vi "SYST_PRES.vi"(0 "VISA IN":refnum<visa-resource-name>, 5 "error in":errorcluster) -> (14 "VISA Out":refnum<visa-resource-name>, 19 "error out":errorcluster)   [LabVIEW 2018, in "PNA-X.lvlib"] (continued)
D6C-00108334AE96}\" \nQuery Syntax Not Applicable \nDefault Not Applicable \nSENSe:CORRection:COLLect:GUIDed:DMATch:APPLy:PORTs? \n1649\n\n(Read-only) Returns the port numbers for which delta match correction is required. 0 (zero) is \nreturned if the Cal does NOT require Delta Match correction for one of the following reasons: \nThe Cal does NOT involve Unknown THRU or TRL. You specify this using \nSENS:CORR:COLL:GUID:METH <UNKN | TRL>. \nThe Cal DOES involve Unknown THRU or TRL, but the delta match data can be calculated by the Unknown \nThru or TRL Cal. Learn how this is possible. However, you can force the Cal to use the Delta Match data \nfrom a Cal Set. \nLearn more about Delta match calibration. \nSee example of a complete Delta Match calibration. \nParameters \nExamples SENS:CORR:COLL:GUID:APPL:PORT? \n'Returns: \n1,2,3 \nReturn Type Numeric \nDefault Not Applicable \nSENSe:CORRection:COLLect:GUIDed:DMATch[:INITiate] <conn>,<cKit> \n(Write-only) Initiates a global delta match calibration. \nLearn more about Global Delta Match calibration. \nSee example of a complete Delta Match calibration. \nParameters \n<conn> String. Connector type for port 1. All other ports are set automatically. \n<cKit> String Cal Kit for all ports. If incorrectly entered while writing, an error is \nreturned. \nExamples SENS:CORR:COLL:GUID:DMAT APC 3.5 female,\"85052B\" \nQuery Syntax Not Applicable \nDefault Not Applicable \nSENSe:CORRection:COLLect:GUIDed:ETERms:LOAD[:CSET] <cset>,<calPort> [,csPort] \n1650\n\n(Write-only) Loads 1-port error terms from a Cal Set into the current Guided Cal sequence. When the \nCal steps are recomputed, connection steps are removed due to the loading of the error terms. \nSee example of how to use this command. \nParameters \n<cset> String Name of User Cal Set in which the error terms reside. \n<pnum> Integer Port number of the current cal to receive error terms. \n[csPort] Integer Optional argument. Port number associated with the error terms in the \nCal Set. If unspecified, the same port number as <calPort> is used. \nExamples See example \nQuery Syntax Not Applicable \nDefault Not Applicable \nSENSe<cnum>:CORRection:COLLect:GUIDed:INITiate [cal set name or GUID [,bool]] \n(Write-only) Initiates a guided calibration. \nThe PNA determines the measurements needed to perform the calibration using the settings specified from \nthe SENS:CORR:COLL:GUID:CONN:PORT and SENS:CORR:COLL:GUID:CKIT:PORT commands. \nAfter this command is executed, subsequent commands can be used to query the number of measurement \nsteps, issue the acquisition commands, query the connection description strings, and subsequently \ncomplete a guided calibration. \nParameters \n<cnum> Any existing channel number. If unspecified, value is set to 1 \n<cal set name or \nGUID> \n(String) Optional argument. If NOT specified, behavior depends on the \nSENS:CORR:PREFerence:CSET:SAVE setting. \nIf specified, choose an existing Cal Set, either by name or by GUID. \nCal Set name including quotes \nCalset GUID in the form: \"{GUID}\"; including quotes and curly brackets. \nQuery all Cal Set GUIDs with SENS:CORR:CSET:CAT? \nSENS:CORR:COLL:GUID:SAVE:CSET can be used instead of this optional \nargument to specify the GUID for a Cal Set. \nAn error is reported if the Cal Set is not found. \n1651\n\nThe Cal Set is either supplemented or overwritten depending on the method, \nconnectors, and ports selected. Learn more about Cal Sets. \n<bool> Optional argument. \nFalse (0) If Cal Set stimulus settings differ from the existing channel, do not \nchange channel stimulus settings. The Cal Set is save to the current setting of \nthe SENS:CORR:PREF:CSET:SAVE command. This is the default setting if \nnot specified. \nTrue (1) If cal set stimulus settings differ from the existing channel, change \nthe channel stimulus settings to match the Cal Set settings. \nExamples SENS:CORR:COLL:GUID:INIT \"{2B893E7A-971A-11d5-8D6C- \n00108334AE96}\",1 \nsense2:correction:collect:guided:initiate 'myCalSet' \nQuery Syntax Not Applicable \nDefault Not Applicable \nSENSe:CORRection:COLLect:GUIDed:ISOLation:AVERage:INCRement <num> \n(Read-Write) Specifies amount to increment (increase) the channel�s averaging factor during \nmeasurement of isolation standards in a guided calibration. \nNote: If the channel has averaging turned OFF and the value of <num> is greater than 1, averaging \nwill be turned ON only during the isolation measurements and with the averaging factor equal to \n<num>.\nParameters \n<num> Amount to increment the averaging factor for the isolation measurement. The \nmaximum averaging factor for the channel is 65536 (2^16). \nExamples 'Measure isolation on all paths for the cal \nSENS:CORR:COLL:GUID:ISOL ALL \n'Remove the port pairs 1-to-2 and 1-to-3 from the list of paths \non which to measure isolation \nsense:correction:collect:guided:isolation:paths REMove,1,2,1,3 \nQuery Syntax SENSe:CORRection:COLLect:GUIDed:ISOLation:PATHs? \nNote: if isolation is not measured, the query returns 0. \nReturn Type Numeric \n1652\n\nDefault 8 - If this command is NOT sent, but isolation is measured, then averaging will \nbe turned ON with factor set to 8 during the isolation measurements. \nSENSe:CORRection:COLLect:GUIDed:ISOLation[:PATHs] <char>[,<p1a, p1b, p2a, p2b,�>] \n(Read-Write) Specifies the paths (port pairs) to make isolation measurements on during a guided \ncalibration. \nParameters \n<char> ALL � Measure isolation on all pairings of the ports that are to be calibrated. \nNONE � Do not measure isolation on any pairing of the ports to be calibrated. \n(Default behavior). \nADD � Add one or more specific pairings of ports to the list of port pairings \nfor which isolation will be measured. \nREMove � Remove one or more specific pairings of ports from the list of port \npairings for which isolation will be measured. If many paths are to be \nmeasured, it may be easier to first send ALL, then REMove and specify the \npaths to remove. \n<p1a, p2a...> For use when <char> is ADD or REMove. \nSpecify Port numbers in pairs: \nFor 3-port cals, specify up to 3 pairs. \nFor 4-port cals, specify up to 6 pairs. \np1a, p1b (Path1 - port A and port B) \np2a, p2b (Path2 - port A and port B) \np3a, p3b (Path3 - port A and port B) \nExamples 'Measure isolation on all paths for the cal \nSENS:CORR:COLL:GUID:ISOL ALL \n'Remove the port pairs 1-to-2 and 1-to-3 from the list of paths \non which to measure isolation \nsense:correction:collect:guided:isolation:paths REMove,1,2,1,3 \n1653\n\nQuery Syntax SENSe:CORRection:COLLect:GUIDed:ISOLation:PATHs? \nNote: if isolation is not be measured on any of the paths, the query returns 0 \nReturn Type Numeric \nDefault 0 - Isolation not measured on any paths. \nSENSe:CORRection:COLLect:GUIDed:METHod <char> Superseded \nThis command is replaced with SENS:CORR:COLL:GUID:PATH:CMEThod and \nSENS:CORR:COLL:GUID:PATH:TMEThod. \n(Read-Write) Selects from one of several algorithms available for performing the THRU portion of a \nguided calibration. Learn more about THRU methods. \nParameters \n<char> DEFAULT - Informs guided calibrations to use the default algorithm when \ncomputing the number of needed standards acquisition steps. (default selection \nif omitted.) \nADAP - Use the adapter removal algorithm \nFLUSH - Use with insertable devices. \nUNKN - Use the Unknown THRU algorithm with calibrations for noninsertable \ndevices. \nDEFined - Use the THRU definition that you stored in the cal kit file, or ECal \nmodule. \nTRL - Select TRL Cal Type for guided cals. Valid for \"TRL ready\" Cal Kits \nwith properly assigned TRL cal classes. \nSOLT - Select SOLT Cal Type for guided cals. Valid for any kit with \nproperly assigned SOLT cal classes. \nExamples SENS:CORR:COLL:GUID:METH ADAP \nsense:correction:collect:guided:method unkn \nQuery Syntax SENSe:CORRection:COLLect:GUIDed:METHod? \nReturn Type Character \nDefault DEFAULT \n1654\n\nSENSe:CORRection:COLLect:GUIDed:PATH:CMEThod \n<port1>,<port2>,<caltype1[,caltype2]> \nNote: This command replaces SENS:CORR:COLL:GUID:METH. \n(Read-Write) Specifies the calibration method for each port pair. \nNote: Before using this command, first do the following: \nSet the connector types: SENS:CORR:COLL:GUID:CONN:PORTn \nSet cal kit: SENS:CORR:COLL:GUID:CKIT:PORT \nSet or query the thru path pairs: SENS:CORR:COLL:GUID:THRU:PORT \nAfter sending or querying this command, send the Thru method: \nSENS:CORR:COLL:GUID:PATH:TMEThod \nParameters \n<port1> First port of the pair to be calibrated. \n<port2> Second port of the pair to be calibrated. \n<caltype1[caltype2]> (String) Cal types for 1st and 2nd ports of the pair, enclosed in a single pair of \nquotes. NOT case-sensitive. \ncaltype1 Cal type for the pair if caltype2 is not specified. Otherwise, Cal type \nfor port 1. Choose from: \n�TRL� \n�SOLT� \n�QSOLTN� \n�EnhRespN \nFor the last two arguments, replace N with the port to be used as the source \nport, which MUST be one of the port pair. \ncaltype2 Optional argument. Use only when performing an adapter removal \ncal on the pair. This argument specifies the Cal type on the second port. \nCaltype1 then specifies the Cal type of the first port. \nChoose from the same arguments as caltype1. \nExamples SENS:CORR:COLL:GUID:PATH:CMEThod 2,3,\"QSOLT2\" \nsense:correction:collect:guided:path:cmethod 2,3,\"solt,trl\" \n1655\n\nQuery Syntax SENSe:CORRection:COLLect:GUIDed:PATH:CMEThod? <port1>,<port2> \nIf only one caltype is returned then it�s NOT adapter removal. \nReturn Type String \nDefault Not Applicable \nSENSe:CORRection:COLLect:GUIDed:PATH:TMEThod \n<port1>,<port2>,<thruType1[,thruType2]> \nNote: This command replaces SENS:CORR:COLL:GUID:METH. \n(Read-Write) Specifies the calibration THRU method for each port pair. \nNote: Before using this command, first do the following: \nSet the connector types: SENS:CORR:COLL:GUID:CONN:PORTn \nSet cal kit: SENS:CORR:COLL:GUID:CKIT:PORT \nSet or query the thru path pairs: SENS:CORR:COLL:GUID:THRU:PORT \nSet or query the Cal Type: SENS:CORR:COLL:GUID:PATH:CMEThod \nLearn more about thru methods. \nParameters \n<port1> First port of the port pair to be calibrated. \n<port2> Second port of the port pair to be calibrated. \n<thruType1[,thruType2]> (String) Thru methods for 1st and 2nd ports of the pair, enclosed in a \nsingle pair of quotes. NOT case-sensitive. \nthruType1 Calibration thru method for the pair if thruType2 is not \nspecified. Otherwise, thru method for port 1. \nChoose from: \n�Defined Thru� A thru type for which there is a stored definition in the Cal \nKit. \n�Zero Thru� Zero length thru, also known as flush-thru. \n�Undefined Thru� A thru type for which there is NOT a stored definition in \nthe Cal Kit. Also known as Unknown Thru. Valid ONLY for SOLT cal type. \n1656\n\n�Undefined Thru using a Defined Thru� Using an ECal module, measure \nthe internal thru using the \"Undefined Thru\" method. \nthruType2 Optional argument. Use only when performing an adapter \nremoval cal on the pair as determined by \nSENS:CORR:COLL:GUID:PATH:CMEThod. The only valid arguments \nfor ThruType1&2 is \"Defined Thru, Defined Thru\". \nExamples SENS:CORR:COLL:GUID:PATH:TMEThod 2,3,�Zero Thru� \nsense:correction:collect:guided:path:tmethod 2,3,\"Defined \nThru,Defined Thru\" \nQuery Syntax SENSe:CORRection:COLLect:GUIDed:PATH:TMEThod \n<port1>,<port2>? \nAlways returns two parts: \nIf the second part of the string is empty, adapter removal is NOT being \nperformed. \nIf the string is \"Defined Thru, Defined Thru\", adapter removal IS being \nperformed. \nReturn Type String \nDefault Not Applicable \nSENSe:CORRection:COLLect:GUIDed:SAVE [bool] \n(Write-only) Completes the guided cal by computing the error correction terms, turning Correction \nON, and saving the calibration to a Cal Set. \nIf all of the required standards have not been measured, the calibration will not complete properly. \nParameters \n[bool] Optional argument. If unspecified, the default behavior is the current PNA \npreference setting of SENSe:CORRection:PREFerence:CSET:SAVE \nFalse (0) Save cal data ONLY to a Cal Register. \nTrue (1) Save cal data to a Cal Register and a User Cal Set. The filename is \nautomatically generated. \nExamples SENS:CORR:COLL:GUID:SAVE \nsense2:correction:collect:guided:save 0 \nQuery Syntax Not Applicable \nDefault Not Applicable \n1657\n\nSENSe:CORRection:COLLect:GUIDed:SAVE:CSET <cal set name or guid> \n(Write-only) Completes the guided cal by computing the error correction terms, turning Correction \nON, and saving the calibration to the specified Cal Set. This command performs the same function as \nSENSe:CORRection:COLLect:GUIDed:SAVE, but this command allows the name or GUID of the \nCal Set to be specified. \nUse this command instead of the optional name or GUID argument in SENS:CORR:COLL:GUID:INIT. \nUse SENS:CORRection:CSET commands to get names or GUIDs of existing Cal Sets. \nThe cal data is also saved to the channel Cal Register. \nIf all of the required standards have not been measured, the calibration will not complete properly. \nParameters \n<cal set name or \nguid> \nString - Name or GUID of an existing Cal Set to be overwritten. If specifying a \nGUID, curly brackets must be included. \nExamples SENS:CORR:COLL:GUID:SAVE:CSET \"{2B893E7A-971A-11d5-8D6C- \n00108334AE96}\" \nsense:correction:collect:guided:save:cset \"MyCalSet\" \nQuery Syntax Not Applicable \nDefault Not Applicable \nSENSe:CORRection:COLLect:GUIDed:STEPs? \n(Read-only) Returns the number of measurement steps required to complete the current guided \ncalibration. This command is sent after the SENS:CORR:COLL:GUID:INIT, \nSENS:CORR:COLL:GUID:CONN:PORT and SENS:CORR:COLL:GUID:CKIT:PORT commands. \nExamples SENS:CORR:COLL:GUID:STEP? \nsense2:correction:collect:guided:steps? \nReturn Type Numeric \nDefault Not Applicable \nSENSe:CORRection:COLLect:GUIDed:THRU:PORTs <t1a, t1b, t2a, t2b, t3a, t3b...> \n1658\n\n(Read-Write) For calibrating more than 2-ports ONLY. Specifies the port pairs for the thru \nconnections of the calibration. \nUse the query to learn the port pairs that the PNA suggests. \nUse the set command to override these thru pairs. \nParameters \n<t1a,...> Specify Port numbers in pairs: \nFor 3-port cals, specify two or three pairs. \nFor 4-port cals, specify from three up to six pairs. \nt1a, t1b (Thru1 - port A and port B) \nt2a, t2b (Thru2 - port A and port B) \nt3a, t3b (Thru3 - port A and port B) \n...and so forth up to six pairs. \nExamples SENS:CORR:COLL:GUID:THRU:PORT 1,2,1,3,1,4 '4-port measurement \nsense:correction:collect:guided:thru:ports 1,2,2,3 '3-port \nmeasurement \nQuery Syntax SENSe:CORRection:COLLect:GUIDed:THRU:PORTs? \nReturn Type Numeric \nDefault Port pairings that were used in the previous cal. \nLast modified: \nApril 14, 2007 Added Cal Set by name and isolation commands \n8-Mar-2007 Added CMethod and TMethod \nOct 23, 2006 Fixed wording in Conn:Port:Sel \n1659\n\nSense:Correction:CKIT Commands \nManages the list of cal kits that are installed in the PNA. \nClick on a blue keyword to view the command details. \nNew See Calibrating the PNA Using SCPI \nLearn about Modifying Cal Kits \nSynchronizing the PNA and Controller \nSCPI Command Tree \nSENSe:CORRection:CKIT:CLEar[:IMMediate] \n(Write-only) Deletes ALL installed cal kits. \nExamples SENS:CORR:CKIT:CLE \nQuery Syntax Not Applicable \nDefault Not Applicable \nSENSe:CORRection:CKIT:COUNt? \n(Read-only) Returns the number of installed cal kits. \nExamples SENS:CORR:CKIT:COUNt? \nQuery Syntax SENS:CORR:CKIT:COUNt? \nReturn Type Numeric \nDefault Not Applicable \n1660\n\nSENSe:CORRection:CKIT:ECAL<mod>:CLISt? \n(Read-only) Returns a list of characterizations stored in the specified ECal module. \nParameters \n<mod> ECal module from which to read user characterization numbers. If unspecified, \nvalue is set to 1. \nExamples Module 1 contains User Characterizations 1 and 3. \nSENSe:CORRection:CKIT:ECAL:CLIST? \n'Returns the following (0 always indicates the factory \ncharacterization): \n0,1,3 \nReturn Type Numeric list, separated by commas. \nDefault Not Applicable \nSENSe:CORRection:CKIT:ECAL<mod>:INFormation? [<char>] \n(Read-only) Reads the user-characterization information from the specified ECal module. This \ncommand returns the same values as SENS:CORR:COLL:CKIT:INF? \nParameters \n<mod> ECal module to read characterizations from. Choose from: \n1 through 8. If unspecified, value is set to 1. \n<char> Optional argument. Specifies which characterization within the ECal module to \nread information from. If not specified, value is set to CHAR0. \nChoose from: \nCHAR0 Factory characterization (data that was stored in the ECal module by \nAgilent) \nCHAR1 User characterization #1 \nCHAR2 User characterization #2 \nCHAR3 User characterization #3 \nCHAR4 User characterization #4 \nCHAR5 User characterization #5 \nExamples SENS:CORR:CKIT:ECAL2:INFormation? char5 \n1661\n\n'Example return string: \nModelNumber: 85092-60007, SerialNumber: 01386, ConnectorType: \nN5FN5F, PortAConnector: Type N (50) female, PortBConnector: Type \nN (50) female, MinFreq: 30000, MaxFreq: 9100000000, \nNumberOfPoints: 250, Calibrated: July 4 2002 \nReturn Type Character \nDefault Not Applicable \nSENSe:CORRection:CKIT:ECAL:LIST? \n(Read-only) Returns a list of index numbers to be used for referring to the ECal modules that are \ncurrently attached to the PNA. \nExamples SENS:CORR:CKIT:ECAL:LIST? \n'If 2 modules are attached to the PNA \n'then the returned list will be: \n1,2 \nReturn Type Numeric list, separated by commas. \nDefault Not Applicable \nSENSe:CORRection:CKIT:ECAL[num]:PATH:COUNt? <path> \n(Read-only) Returns the number of unique states that exist for the specified path name on the selected \nECal module. \nThis command performs exactly the same function as CONT:ECAL:MOD:PATH:COUNt? \nUse the CONT:ECAL:MOD:PATH:STAT command to set the module into one of those states. \nUse SENS:CORR:CKIT:ECAL:PATH:DATA? to read the data for a state. \nParameters \n[num] Optional argument. USB number of the ECal module. If unspecified (only one \nECal module is connected to the USB), <num> is set to 1. If two or more \nmodules are connected, use SENS:CORR:CKIT:ECAL:LIST? to determine \nhow many, and SENS:CORR:CKIT:ECAL:INF? to verify their identities. \n<path> Name of the path for which to read number of states. Choose from: \nReflection paths \n1662\n\nA\nB\nC (4-port modules) \nD (4-port modules) \nTransmission paths \nAB \nAC (4-port modules) \nAD (4-port modules) \nBC (4-port modules) \nBD (4-port modules) \nCD (4-port modules) \nExamples CONT:ECAL:MOD:PATH:COUNt? \ncontrol:ecal:module2:path:count? \nReturn Type Integer \nDefault Not Applicable \nSENSe<ch>:CORRection:CKIT:ECAL[num]:PATH:DATA? <path>, <stateNum>|,<char>| \n(Read-only) Returns the data for a state from the memory of the selected ECal module. The returned \ndata is interpolated if necessary to have the same stimulus values as the specified channel <ch>. \nFor a reflection path state, the data is reflection S-parameter data. The number of values equals the \nnumber of stimulus points on the channel multiplied by 2 (because they are complex numbers). \nFor a transmission path state, the data is all 4 S-parameters of the state. The number of values returned is \n4 times that of a reflection state. \nThe data is returned in the same format as CALC:DATA:SNP? \nNote: This command returns SNP data without header information, and in columns, not in rows as \n.SnP files. This means that the data returned from this command sends all frequency data, then all Sx1 \nmagnitude data, then all Sx1 phase data, and so forth. \nParameters \n<ch> Any existing channel number. If unspecified, value is set to 1. \n1663\n\n[num] Optional argument. USB number of the ECal module. If unspecified (only one \nECal module is connected to the USB), <num> is set to 1. If two or more \nmodules are connected, use SENS:CORR:CKIT:ECAL:LIST? to determine \nhow many, and SENS:CORR:CKIT:ECAL:INF? to verify their identities. \n<path> Name of the path for which to read number of states. Choose from: \nReflection paths \nA\nB\nC (4-port modules) \nD (4-port modules) \nTransmission paths \nAB \nAC (4-port modules) \nAD (4-port modules) \nBC (4-port modules) \nBD (4-port modules) \nCD (4-port modules) \n<stateNum> Number of the state to set. Refer to the following table to associate the \n<stateNum> with a state in your ECal module. \nIn addition, CONT:ECAL:MOD:PATH:COUNt? returns the number of states \nin the specified ECal module. \n1664\n\n<stateNum> N4432A \nand \nN4433A \nStates \nN4431A \nStates \nN469x \nStates** \n8509x \nStates \nOne-Port Reflection States \n1 Open Open Impedance \n1 \nOpen \n2 Short Short Impedance \n2 \nShort \n3 Impedance \n1 \nImpedance \n1 \nImpedance \n3 \nImpedance \n1 \n4 Impedance \n2 \nImpedance \n2 \nImpedance \n4 \nImpedance \n2 \n5 Impedance \n5 \n6 Impedance \n6 \n7 Impedance \n7 \nTwo-Port Transmission States \n1 Thru Thru Thru Thru \n2 Confidence Confidence Confidence Confidence \n** The following modules have only FOUR Impedance states (1, 2, 3, 4): \nN4690B ,N4691B ,N4692A ,N4696B. \n<char> Optional argument. Specifies which characterization within the ECal module to \nread information from. If not specified, value is set to CHAR0. \nChoose from: \nCHAR0 Factory characterization (data that was stored in the ECal module by \nAgilent) \nCHAR1 User characterization #1 \nCHAR2 User characterization #2 \nCHAR3 User characterization #3 \nCHAR4 User characterization #4 \nCHAR5 User characterization #5 \n1665\n\nExamples SENS:CORR:CKIT:ECAL1:PATH:DATA? \nReturn Type S1P or S2P \nDefault Not Applicable \nSENSe:CORRection:CKIT:IMPort <string> \n(Write-only) Imports the specified cal kit (.ckt file) and appends the imported kit to the end of the list \nof kits whenever the file import succeeds. \nParameters \n<string> Path and cal kit name. \nExamples SENSe:CORRection:CKIT:IMPort \"C:/Program Files/Agilent/Network \nAnalyzer/Documents/85033D.ckt\" \nQuery Syntax Not Applicable \nDefault Not Applicable \nSENSe:CORRection:CKIT:INITialize[:IMMediate] \n(Write-only) Restores all default factory installed cal kits. \nParameters \nExamples SENS:CORR:CKIT:INITialize \nsense:correction:ckit:initialize \nQuery Syntax Not Applicable \nDefault Not Applicable \nSENSe:CORRection:CKIT:LOAD <string> \n(Write-only) Loads the specified collection of cal kits from a .wks file. You can make your own \ncollection of cal kits from the Advanced Modify Cal Kit menu. \nParameters \n<string> Path and file name of the cal kit collection. \nExamples sense:correction:ckit:load \"C:/Program Files/Agilent/Network \nAnalyzer/PnaCalKits/factory/wMyCalKits.wks \nQuery Syntax Not Applicable \nDefault Not Applicable \n1666\n\nLast modified: \n10/16/06 Modified Ecal:Data to include <ch> \n1667\n\nSense:Correction:Collect:Ckit Commands \nUse to change the definitions of calibration kit standards. \nClick on a blue keyword to view the command details. \nMost of these commands act on the currently selected standard from the currently selected calibration \nkit. \nTo select a Calibration kit, use SENS:CORR:COLL:CKIT:SEL. \nTo select a Calibration standard, use SENS:CORR:COLL:CKIT:STAN:SEL \nSee an example program that CREATES a New Cal Kit \nSee an example program that MODIFIES an Existing Cal Kit \nLearn about Modifying Cal Kits \nSynchronizing the PNA and Controller \nSCPI Command Tree \nNote: You should provide data for every definition field - for every standard in your calibration kit. If a \nfield is not set, the default value may not be what you expect. \nSENSe:CORRection:COLLect:CKIT:CONNector:ADD \n<family>,<start>,<stop>,<z0>,<gender>,<media>,<cutoff> \n1668\n\n(Write only) Creates a new connector. The connector is automatically added to the list of available \nconnectors for the currently selected cal kit. If a connector includes both male and female connectors, \neach connector must be added separately. \nParameters \n<family> (String) Name of connector family. Limited to 50 characters. \n<start> Start frequency \n<stop> Stop frequency \n<z0> Characteristic Impedance of the connector in ohms. \n<gender> Connector gender. Choose from: \nMALE \nFEMALE \nNONE \n<media> Media of the connector. Choose from: \nCOAX - coaxial \nWAVE - waveguide \n<cutoff> Cutoff frequency of the connector (waveguide only). \nExamples SENS:CORR:COLL:CKIT:CONN:ADD \"PSC 1.8 mm\",0 HZ,999.9 \nGHZ,50,FEMALE,COAX,0.0 \nSENS:CORR:COLL:CKIT:CONN:ADD \"PSC 1.8 mm\",0 HZ,999.9 \nGHZ,50,MALE,COAX,0.0 \nQuery Syntax Not applicable \nDefault Not Applicable \nSENSe:CORRection:COLLect:CKIT:CONNector:CATalog? \n1669\n\n(Read-only) Returns a comma-separated list of all connectors defined within the currently selected cal \nkit. The returned string includes the connector family name followed by the connector gender, if any. \nKits may include a primary connector family name and additional connector family names. \nConnector family names are case sensitive. A connector family named \"PSC 2.4\" is different from a \nconnector family named \"psc 2.4\". \nLearn more about Connector Family Name \nExamples SENS:CORR:COLL:CKIT:CONN:CAT? \n'Returned string \n\"Type-N (50) male, Type-N (50) female\" \nDefault Not Applicable \nSENSe:CORRection:COLLect:CKIT:CONNector:DELete \n(Write-only) Deletes the primary connector family name from the selected kit. The PNA allows \nmultiple connector families for each kit. If a kit includes multiple connector families, only the first \nlisted (primary) connector family name is deleted. \nOnce the connector family is deleted, the connector may not be assigned to any new or existing \nstandard within the kit. \nThe previously defined standards retain their association to the deleted connector name. To reassign \nstandards to a new connector family name, use SENS:CORR:COLL:CKIT:CONN:SNAMe. \nExamples SENS:CORR:COLL:CKIT:CONN:DEL \nQuery Syntax Not Applicable \nDefault Not Applicable \nSENSe:CORRection:COLLect:CKIT:CONNector:FNAME <name> \n1670\n\n(Read-Write) Replaces the primary connector family name from the selected kit with a new connector \nfamily name. The connector family name is replaced in all standards in the kit that share that name. \nThe PNA allows multiple connector families for each kit. If a kit includes multiple connector \nfamilies, only the first listed (primary) connector family name is replaced. Use the query form of this \ncommand to return the name of the primary connector family. \nParameters \n<name> New connector family name. Limited to 50 characters. \nExamples SENS:CORR:COLL:CKIT:CONN:FNAM 'MYPSC35' \nSense:correction:collect:ckit:connector:name 'My Type N' \nQuery Syntax SENSe:CORRection:COLLect:CKIT:CONNector:FNAMe? \nReturn Type String \nDefault Not Applicable \nSENSe:CORRection:COLLect:CKIT:CONNector:SNAMe <family>,<gender>,<port> \n(Read-Write) Assigns a family name to the currently selected standard from the currently selected kit. \nSpecify each port of a 2-port standard individually. Use the query form of this command to read the \nconnector family name assigned to the current standard. The name is not assigned unless the \nconnector family name is previously defined within the selected kit. \nParameters \n<family> String. Connector family name. \n<gender> Connector gender. Choose from: \nMALE \nFEMALE \nNONE \n<port> Number of the connector port to be assigned the connector family name. 2-port \nstandards such as a thru line must be assigned separately. It is not relevant \nwhich connector is port 1 or port 2. \n1 Specifies a 1-port standard or the first port of a 2-port standard. \n2 Specifies the second port of a 2-port standard. \nExamples SENS:CORR:COLL:CKIT:CONN:SNAMe \"Type-N (50)\",MALE,1 \nQuery Syntax SENSe:CORRection:COLLect:CKIT:CONNector:SNAMe? \nReturn Type String \n1671\n\nDefault Not Applicable \nSENSe:CORRection:COLLect:CKIT:DESCription <string> \n(Read-Write) Modifies the cal kit description field of the selected kit. This description appears in the \nEdit PNA Cal Kit dialog box. \nParameters \n<string> Description of the cal kit. Limited to 50 characters. \nExamples SENS:CORR:COLL:CKIT:DESC \"My New CalKit\" \nQuery Syntax SENSe:CORRection:COLLect:CKIT:DESCription? \nReturn Type String \nDefault Not Applicable \nSENSe:CORRection:COLLect:CKIT:INFormation? <module>[,char] \n(Read Only) Reads characterization information from an ECal module. \nParameters \n<module> Specifies which ECal module to read from. Choose from: \nECAL1 \n.through. \nECAL8 \n[char] \nOptional argument. \nSpecifies which characterization within the ECal module to read information \nfrom. If this argument is not used, the default is CHAR0. CHAR1 through \nCHAR5 are for user characterizations that may have been written to the \nmodule by the User Characterization feature on the PNA. Choose from: \nCHAR0 Factory characterization (data that was stored in the ECal module by \nAgilent) \nCHAR1 User characterization #1 \nCHAR2 User characterization #2 \nCHAR3 User characterization #3 \n1672\n\nCHAR4 User characterization #4 \nCHAR5 User characterization #5 \nExamples SENS:CORR:COLL:CKIT:INF? ECAL4 \nsense:correction:collect:ckit:information? ecal2,char1 \nExample return string: \nModelNumber: 85092-60007, SerialNumber: 01386, ConnectorType: \nN5FN5F, PortAConnector: Type N (50) female, PortBConnector: Type \nN (50) female, MinFreq: 30000, MaxFreq: 9100000000, \nNumberOfPoints: 250, Calibrated: July 4 2002 \nReturn Type Character \nDefault Not Applicable \nSENSe:CORRection:COLLect:CKIT:NAME <name> \n(Read-Write) Sets a name for the selected calibration kit. \nParameters \n<name> Calibration Kit name. Any string name, can include numerics, period, and \nspaces; any length (although the dialog box display is limited to about 30 \ncharacters). \nExamples SENS:CORR:COLL:CKIT:NAME 'MYAPC35' \nsense:correction:collect:ckit:name 'mytypen' \nQuery Syntax SENSe:CORRection:COLLect:CKIT:NAME? \nReturn Type String \nDefault Not Applicable \nSENSe:CORRection:COLLect:CKIT:OLABel<class> <name> \n(Read-Write) Sets the label for the calibration class designated by <class>. The label is used in the \nprompts for connecting the calibration standards associated with that <class>. \nParameters \n<class> Number of the calibration class. Choose a number between: 1 and 18. The \n<class> numbers are associated with the following calibration Classes: \n1673\n\nClass Description \n1 S11A Reflection standard \n2 S11B Reflection standard \n3 S11C Reflection standard \n4 S21T Thru/Delay standard \n5 S22A Reflection standard \n6 S22B Reflection standard \n7 S22C Reflection standard \n8 S12T Thru/Delay standard \n3-port analyzers only \n9 S33A Reflection standard \n10 S33B Reflection standard \n11 S33C Reflection standard \n12 S32T Thru/Delay standard \n13 S23T Thru/Delay standard \n14 S31T Thru/Delay standard \n15 S13T Thru/Delay standard \nTRL Calibrations \n16 TRL \"T\" Thru standard \n17 TRL \"R\" Reflect standard \n18 TRL \"L\" Line standard \n<name> Label for the calibration class. Must be enclosed in quotes. Any string \nbetween 1 and 12 characters long. Cannot begin with a numeric. \nExamples SENS:CORR:COLL:CKIT:OLAB3 'LOADS' \nsense:correction:collect:ckit:olabel4 'Thru' \nReturn Type String \nDefault Not Applicable \nSENSe:CORRection:COLLect:CKIT:OLIST[class]? \n(Read-only) Returns seven values of standards that are assigned to the specified class. \nParameters \n<class> Number of the calibration class to be queried. The <class> numbers are \nassociated with the following calibration Classes: \n1674\n\nClass Description \n1 S11A Reflection standard \n2 S11B Reflection standard \n3 S11C Reflection standard \n4 S21T Thru/Delay standard \n5 S22A Reflection standard \n6 S22B Reflection standard \n7 S22C Reflection standard \n8 S12T Thru/Delay standard \n3-port analyzers ONLY \n4-port analyzers use S11 and S22 classes (see example program) \n9 S33A Reflection standard \n10 S33B Reflection standard \n11 S33C Reflection standard \n12 S32T Thru/Delay standard \n13 S23T Thru/Delay standard \n14 S31T Thru/Delay standard \n15 S13T Thru/Delay standard \nTRL Calibrations \n16 TRL \"T\" Thru standard \n17 TRL \"R\" Reflect standard \n18 TRL \"L\" Thru standard \nExamples SENS:CORR:COLL:CKIT:OLIST8? \nAlways returns 7 standard numbers. Unassigned standards return 0 \nReturn Type Numeric; returns the <class> number of the selected standard. \nDefault Not Applicable \nSENSe:CORRection:COLLect:CKIT:ORDer<class> <std> [,<std>] [,<std>] [,<std>] [,<std>] \n[,<std>] [,<std>] \n1675\n\n(Read-Write) Sets a standard number to a calibration class. Does NOT set or dictate the order for \nmeasuring the standards. For more information, see Assigning Standards to a Calibration Class \nParameters \n<class> Number of the calibration class that is assigned to <standard>. Choose a \nnumber between: 1 and 18. The <class> numbers are associated with the \nfollowing calibration Classes: \nClass Description \n1 S11A Reflection standard \n2 S11B Reflection standard \n3 S11C Reflection standard \n4 S21T Thru/Delay standard \n5 S22A Reflection standard \n6 S22B Reflection standard \n7 S22C Reflection standard \n8 S12T Thru/Delay standard \n3-port analyzers ONLY \n4-port analyzers use S11 and S22 classes (see example program) \n9 S33A Reflection standard \n10 S33B Reflection standard \n11 S33C Reflection standard \n12 S32T Thru/Delay standard \n13 S23T Thru/Delay standard \n14 S31T Thru/Delay standard \n15 S13T Thru/Delay standard \nTRL Calibration \n16 TRL \"T\" Thru standard \n17 TRL \"R\" Reflect standard \n18 TRL \"L\" Line standard \n1676\n\n<std> Standard number to be assigned to the class; Choose a standard between 1 and \n8. One standard is mandatory; up to six additional standards are optional. \nExamples Assigns standard 3 to S11A class: \nSENS:CORR:COLL:CKIT:ORD1 3 \nAssigns standard 2 and 5 to S21T class class: \nsense:correction:collect:ckit:order4 2,5 \nQuery Syntax SENSe:CORRection:COLLect:CKIT:ORDer<class>? \n'Returns only the first standard assigned to the specified class. To \nquery the remaining standards, use \nSENSe:CORRection:COLLect:CKIT:OLIST[1-15]? \nReturn Type Numeric \nDefault Not Applicable \nSENSe:CORRection:COLLect:CKIT:RESet <num> - Superseded \nThis command is replaced by Sens:Corr:Ckit:Init. \n(Write-only) Resets the selected calibration kit to factory default definition values. \nParameters \n<num> The number of the calibration kit to be reset. Choose any integer between: \n1 and 8 \nExamples SENS:CORR:COLL:CKIT:RESet 1 \nsense:correction:collect:ckit:reset 4 \nQuery Syntax Not Applicable \nDefault Not Applicable \nSENSe:CORRection:COLLect:CKIT[:SELect] <num> \n1677\n\n(Read-Write) Selects (makes active) a calibration kit for performing a calibration or for modifying \nstandards. All subsequent \"CKIT\" commands that are sent apply to this selected calibration kit. Select \na calibration standard using SENS:CORR:COLL:CKIT:STAN <num> \nParameters \n<num> The number of the calibration kit. Choose from: \nUse SENSe:CORRection:COLLect:CKIT:RESet to restore Cal Kits to default \nvalues. \nName \n1 User Defined 1 \n2 User Defined 2 \n3 User Defined 3 \n'' \n'' \n48 User Defined 48 \n49 User Defined 49 \n50 User Defined 50 \n99 ECAL module \nExamples SENS:CORR:COLL:CKIT 2 \nsense2:correction:collect:ckit:select 7 \nQuery Syntax SENSe:CORRection:COLLect:CKIT? \nReturn Type Numeric \nDefault Last kit selected \nSENSe:CORRection:COLLect:CKIT:STANdard:C0 <num> \n1678\n\n(Read-Write) Sets the C0 value (the first capacitance value) for the selected standard. For a detailed \ndiscussion of this value, search for App Note 8510-5B at www.Agilent.com. \nParameters \n<num> Value for C0 in femtofarads (1E-15) \nExamples The following commands set C0=15 femtofarads: \nSENS:CORR:COLL:CKIT:STAN:C0 15 \nsense:correction:collect:ckit:standard:c0 15 \nQuery Syntax SENSe:CORRection:COLLect:CKIT:STANdard:C0? \nReturn Type Numeric \nDefault Not Applicable \nSENSe:CORRection:COLLect:CKIT:STANdard:C1 <num> \n(Read-Write) Sets the C1 value (the second capacitance value) for the selected standard. For a detailed \ndiscussion of this value, search for App Note 8510-5B at www.Agilent.com. \nParameters \n<num> Value for C1. \nExamples The following two commands set C1=15: \nSENS:CORR:COLL:CKIT:STAN:C1 15 \nsense:correction:collect:ckit:standard:c1 15 \nQuery Syntax SENSe:CORRection:COLLect:CKIT:STANdard:C1? \nReturn Type Numeric \nDefault Not Applicable \nSENSe:CORRection:COLLect:CKIT:STANdard:C2 <num> \n1679\n\n(Read-Write) Sets the C2 value (the third capacitance value) for the selected standard. For a detailed \ndiscussion of this value, search for App Note 8510-5B at www.Agilent.com. \nParameters \n<num> Value for C2. \nExamples The following two commands set C2: \nSENS:CORR:COLL:CKIT:STAN:C2 15 \nsense:correction:collect:ckit:standard:c2 15 \nQuery Syntax SENSe:CORRection:COLLect:CKIT:STANdard:C2? \nReturn Type Numeric \nDefault Not Applicable \nSENSe:CORRection:COLLect:CKIT:STANdard:C3 <num> \n(Read-Write) Sets the C3 value (the fourth capacitance value) for the selected standard. For a detailed \ndiscussion of this value, search for App Note 8510-5B at www.Agilent.com. \nParameters \n<num> Value for C3. \nExamples The following two commands set C3 \nSENS:CORR:COLL:CKIT:STAN:C3 15 \nsense:correction:collect:ckit:standard:c3 15 \nQuery Syntax SENSe:CORRection:COLLect:CKIT:STANdard:C3? \nReturn Type Numeric \nDefault Not Applicable \nSENSe:CORRection:COLLect:CKIT:STANdard:CHARacter <char> \n1680\n\n(Read-Write) Sets the media type of the selected calibration standard. \nParameters \n<char> Media type of the standard. Choose from: \nCoax - Coaxial Cable \nWave - Waveguide \nExamples SENS:CORR:COLL:CKIT:STAN:CHAR COAX \nsense:correction:collect:ckit:standard:character wave \nQuery Syntax SENSe:CORRection:COLLect:CKIT:STANdard:CHARacter? \nReturn Type Numeric \nDefault Coax \nSENSe:CORRection:COLLect:CKIT:STANdard:DELay <num> \n(Read-Write) Sets the electrical delay value for the selected standard. \nParameters \n<num> Electrical delay in picoseconds \nExamples The following two commands set delay to 50 picoseconds \nSENS:CORR:COLL:CKIT:STAN:DEL 50e-12 \nsense2:correction:collect:ckit:standard:delay 50ps \nQuery Syntax SENSe:CORRection:COLLect:CKIT:STANdard:DELay? \nReturn Type Numeric \nDefault Not Applicable \nSENSe:CORRection:COLLect:CKIT:STANdard:FMAX <num> \n1681\n\n(Read-Write) Sets the maximum frequency for the selected standard. \nParameters \n<num> Maximum frequency in Hertz. \nExamples SENS:CORR:COLL:CKIT:STAN:FMAX 9e9 \nsense:correction:collect:ckit:standard:fmax 9Ghz \nQuery Syntax SENSe:CORRection:COLLect:CKIT:STANdard:FMAX? \nReturn Type Numeric \nDefault Not Applicable \nSENSe:CORRection:COLLect:CKIT:STANdard:FMIN <num> \n(Read-Write) Sets the minimum frequency for the selected standard. \nParameters \n<num> Minimum frequency in Hertz. \nExamples SENS:CORR:COLL:CKIT:STAN:FMIN 1e3 \nsense:correction:collect:ckit:standard:fmin 1khz \nQuery Syntax SENSe:CORRection:COLLect:CKIT:STANdard:FMIN? \nReturn Type Numeric \nDefault Not Applicable \nSENSe:CORRection:COLLect:CKIT:STANdard:IMPedance <num> \n(Read-Write) Sets the characteristic impedance for the selected standard. \nParameters \n<num> Impedance in Ohms \nExamples SENS:CORR:COLL:CKIT:STAN:IMP 75 \nsense:correction:collect:ckit:standard:impedance 50.3 \nQuery Syntax SENSe:CORRection:COLLect:CKIT:STANdard:IMPedance? \nReturn Type Numeric \nDefault 50 \nSENSe:CORRection:COLLect:CKIT:STANdard:L0 <num> \n1682\n\n(Read-Write) Sets the L0 value (the first inductance value) for the selected standard. For a detailed \ndiscussion of this value, search for App Note 8510-5B at www.Agilent.com. \nParameters \n<num> Value for L0 in femtohenries (1E-15) \nExamples The following two commands set L0=15 femtohenries: \nSENS:CORR:COLL:CKIT:STAN:L0 15 \nsense:correction:collect:ckit:standard:l0 15 \nQuery Syntax SENSe:CORRection:COLLect:CKIT:STANdard:L0? \nReturn Type Numeric \nDefault Not Applicable \nSENSe:CORRection:COLLect:CKIT:STANdard:L1 <num> \n(Read-Write) Sets the L1 value (the second inductance value) for the selected standard. For a detailed \ndiscussion of this value, search for App Note 8510-5B at www.Agilent.com. \nParameters \n<num> Value for L1. \nExamples The following two commands set L1=15: \nSENS:CORR:COLL:CKIT:STAN:L1 15 \nsense:correction:collect:ckit:standard:l1 15 \nQuery Syntax SENSe:CORRection:COLLect:CKIT:STANdard:L1? \nReturn Type Numeric \nDefault Not Applicable \nSENSe:CORRection:COLLect:CKIT:STANdard:L2 <num> \n1683\n\n(Read-Write) Sets the L2 value (the third inductance value) for the selected standard. For a detailed \ndiscussion of this value, search for App Note 8510-5B at www.Agilent.com. \nParameters \n<num> Value for L2. \nExamples The following two commands set L2=15: \nSENS:CORR:COLL:CKIT:STAN:L2 15 \nsense:correction:collect:ckit:standard:l2 15 \nQuery Syntax SENSe:CORRection:COLLect:CKIT:STANdard:L2? \nReturn Type Numeric \nDefault Not Applicable \nSENSe:CORRection:COLLect:CKIT:STANdard:L3 <num> \n(Read-Write) Sets the L3 value (the fourth inductance value) for the selected standard. For a detailed \ndiscussion of this value, search for App Note 8510-5B at www.Agilent.com. \nParameters \n<num> Value for L3. \nExamples The following two commands set L3=15: \nSENS:CORR:COLL:CKIT:STAN:L3 15 \nsense:correction:collect:ckit:standard:l3 15 \nQuery Syntax SENSe:CORRection:COLLect:CKIT:STANdard:L3? \nReturn Type Numeric \nDefault Not Applicable \nSENSe:CORRection:COLLect:CKIT:STANdard:LABel <name> \n1684\n\n(Read-Write) Sets the label for the selected standard. The label is used to prompt the user to connect \nthe specified standard. \nParameters \n<name> Label for the standard; Must be enclosed in quotes. Any string between 1 and \n12 characters long. Cannot begin with a numeric. \nExamples SENS:CORR:COLL:CKIT:STAN:LAB 'OPEN' \nsense:correction:collect:ckit:standard:label 'Short2' \nQuery Syntax SENSe:CORRection:COLLect:CKIT:STANdard:LABel? \nReturn Type String \nDefault Not Applicable \nSENSe:CORRection:COLLect:CKIT:STANdard:LOSS <num> \n(Read-Write) Sets the insertion loss for the selected standard. \nParameters \n<num> Insertion loss in Gohms / sec. (GigaOhms per second of electrical delay) \nExamples SENS:CORR:COLL:CKIT:STAN:LOSS 3.5e9 \nsense:correction:collect:ckit:standard:loss 3 \nQuery Syntax SENSe:CORRection:COLLect:CKIT:STANdard:LOSS? \nReturn Type Numeric \nDefault Not Applicable \nSENSe:CORRection:COLLect:CKIT:STANdard:REMove \n(Write only) Deletes the selected standard from the selected cal kit. \nExamples SENS:CORR:COLL:CKIT:STAN:REMove \nDefault Not Applicable \nSENSe:CORRection:COLLect:CKIT:STANdard:SDEScription <string> \n1685\n\n(Read-Write) Modifies the description of the selected standard of the selected kit. This description \nappears in the edit kit dialog box. \nParameters \n<string> Description of the standard. \nExamples SENS:CORR:COLL:CKIT:STAN:SDES \"My New Standard\" \nQuery Syntax SENSe:CORRection:COLLect:STANdard:SDEScription? \nReturn Type String \nDefault Not Applicable \nSENSe:CORRection:COLLect:CKIT:STANdard[:SELECT] <num> \n(Read-Write) Selects the calibration standard. All subsequent \"CKIT\" commands to modify a standard \nwill apply to the selected standard. Select a calibration kit using SENS:CORR:COLL:CKIT:SEL \nParameters \n<num> Number of the standard. Choose any number between: \n1 and 30 \nExamples SENS:CORR:COLL:CKIT:STAN 3 \nsense:correction:collect:ckit:standard:select 8 \nQuery Syntax SENSe:CORRection:COLLect:CKIT:STANdard[:SELect]? \nReturn Type Numeric \nDefault 1 \nSENSe:CORRection:COLLect:CKIT:STANdard:TYPE <char> \n1686\n\n(Read-Write) Sets the type for the selected standard. \nParameters \n<char> Choose from: \nOPEN \nSHORT \nLOAD \nSLOAD (sliding load) \nTHRU (through) \nARBI(arbitrary) \nExamples SENS:CORR:COLL:CKIT:STAN:TYPE LOAD \nsense:correction:collect:ckit:standard:type short \nQuery Syntax SENSe:CORRection:COLLect:CKIT:STANdard:TYPE? \nReturn Type Character \nDefault Not Applicable \nSENSe:CORRection:COLLect:CKIT:STANdard:TZReal <num> \n(Read-Write) Sets the TZReal component value of the Terminal Impedance for the selected standard. \nNote: Only applicable when the Standard Type is set to ARBI \nParameters \n<num> Value for TZReal in Ohms \nExamples The following commands set TZReal=15 Ohms: \nSENS:CORR:COLL:CKIT:STAN:TZReal 15 \nsense:correction:collect:ckit:standard:TZReal 15 \nQuery Syntax SENSe:CORRection:COLLect:CKIT:STANdard:TZReal? \nReturn Type Numeric \nDefault Not Applicable \nSENSe:CORRection:COLLect:CKIT:STANdard:TZImag <num> \n1687\n\n(Read-Write) Sets the TZImag component value of the Terminal Impedance for the selected standard. \nNote: Only applicable when the Standard Type is set to ARBI \nParameters \n<num> Value for TZImag in Ohms \nExamples The following two commands set TZImag=15 Ohms: \nSENS:CORR:COLL:CKIT:STAN:TZImag 15 \nsense:correction:collect:ckit:standard:TZImag 15 \nQuery Syntax SENSe:CORRection:COLLect:CKIT:STANdard:TZImag? \nReturn Type Numeric \nDefault Not Applicable \n1688\n\nSense:Correction:Cset Commands \nPerforms actions on calibration sets. \nClick on a blue keyword to view the command details. \nSee Also \nCreating Cal Sets \nExample Programs \nLearn about Cal Sets \nSynchronizing the PNA and Controller \nSENSe<cnum>:CORRection:CSET:ACTivate <string>, <bool> \nThis command replaces SENS:CORR:CSET:GUID \n(Read-Write) Selects and applies a Cal Set to the specified channel. \nUse SENS:CORR:CSET:CAT? to list the Cal Sets. \nParameters \n<cnum> Any existing channel number. If unspecified, value is set to 1 \n<string> Cal Set to make active. Specify the Cal Set by GUID or Name. Use \nSENS:CORR:CSET:CAT? to list the available Cal Sets in either format. \n<bool> Should the Cal Set stimulus values be applied to the channel. Choose from: \nON (1) Apply the Cal Set stimulus values to the channel. \nOFF (0) Do NOT apply the Cal Set stimulus values. If the Cal Set stimulus \nvalues do not match the channel stimulus values, then the following will occur: \n1689\n\nIf interpolation is ON, then interpolation will be attempted. This may fail if the \nchannel frequency is outside the range of the Cal Set. \nIf interpolation is OFF, the selection will be abandoned and an error is returned: \nExamples SENS:CORR:CSET:ACT \"My2Port\",1 \nsense:correction:cset:activate? name \n'returns \n\"My2Port\" \nQuery Syntax SENSe<cnum>:CORRection:CSET:ACTivate? [GUID|NAME] \nReturns the name of the Cal Set that is applied to the specified channel. Choose \nfrom GUID or NAME to specify which string is returned. If unspecified, the \nGUID of the Cal Set is returned. If no Cal Set is applied to the specified \nchannel, then \"No Calset Selected\" is returned. \nReturn Type String \nDefault Not Applicable \nSENSe:CORRection:CSET:CATalog? [char] \n(Read-only) Returns a list of Cal Sets. \nParameters \n<char> Optional argument. The list is returned in one of the following formats. Both \nreturn comma-separated string lists. \nGUID Cal Sets are listed by GUID (Default if unspecified). \nNAME Cal Sets are listed by Name \nExamples SENS:CORR:CSET:CAT? \n'Returns: \n{FD6F863E-9719-11d5-8D6C-00108334AE96},{1B03B2CE-971A-11d5-8D6C- \n00108334AE96} \nsense2:correction:cset:catalog? name \nDefault Not Applicable \nSENSe<cnum>:CORRection:CSET:CREate [name] \n1690\n\n(Write-only) Creates an empty Cal Set and attaches it to the specified channel. This command is \nONLY necessary before remotely filling the Cal Set with error term data. (For Advanced Users). \nA Cal Set is automatically created, applied to the channel, and saved at the completion of a guided cal \naccording to the preference setting SENS:CORR:PREF:CSET:SAVE. \nParameters \n<cnum> Any existing channel number. If unspecified, value is set to 1 \n[name] Optional argument. Name of the Cal Set. Spaces or punctuation are NOT \nallowed. If unspecified, a unique name is chosen in the form \"Calset_N\" where \nN is a unique number. \nExamples SENS:CORR:CSET:CRE 'My2Port' \nQuery Syntax Not Applicable \nDefault Not Applicable \nSENSe<cnum>:CORRection:CSET:DATA <eterm, portA, portB,>[<param>,] <block> \n(Read-Write) Read or Write a specific error term from/to the Cal Set currently attached to the \nspecified channel. (For Advanced Users). \nParameters \n<cnum> Any existing channel number. If unspecified, value is set to 1 \n<eterm, portA, \nportB> \nError Term, Port pair of the specified error term. \nAlthough not all error terms use two port numbers, two are required by the \nPNA in all cases. Each port number must be between 1 and the number of ports \non the PNA. \nEDIR - directivity \nportA: the port at which directivity is measured \nportB: Not used, but must be a valid PNA port number. \nESRM - source match \nportA: the port at which source match is measured \nportB: Not used, but must be a valid PNA port number. \n1691\n\nERFT - reflection tracking \nportA: the port at which reflection tracking is measured \nportB: Not used, but must be a valid PNA port number. \nELDM - load match \nportA: the port at which load match is measured \nportB: the source port. \nLoad match is measured with a cable connected between the measured port \n(portA) and the source port (portB). \nThe cal system requires that the complete matrix of loadmatch arrays be filled. \nIn most cases you can measure loadmatch once at a port, driven by any other \nport. Then use that data for all variations of the receive port. (The exception is \nthe 3-port PNA models, which requires the loadmatch-measured port to be \ndriven by every other port.) \nFor example: Measure the loadmatch at port2 while driving port1. Then upload \nthis same data to the following arrays: \nELDM,2,1,<data> \nELDM,2,3,<data> \nELDM,2,4,<data> \nETRT - transmission tracking \nportA: the receive port \nportB: the source port for this measurement \nEXTLK - crosstalk \nportA: the receive port \nportB: the source port for this measurement \nERSPT - response tracking. \nportA: Not used, but must be a valid PNA port number. \nportB: Not used, but must be a valid PNA port number. \n1692\n\nERSPI - response isolation. \nportA: Not used, but must be a valid PNA port number. \nportB: Not used, but must be a valid PNA port number. \n<param> <string> - required ONLY when Eterm is response tracking (ERSPT) or \nresponse isolation (ERSPI). Specify the S-parameter, ratio, or unratioed \nmeasurement for which the Eterm applies. \nLogical receiver notation is allowed. Ratioed measurements do not require \nsource port to be specified. \nA full 4-port calibration requires the following terms be uploaded: \nPORT B \n1 2 3 4 \nP\nO\nR\nT \nA \n1 \nEDIR,1,1 \nERFT,1,1 \nESRM,1,1 \nELDM,1,2 \nETRT,1,2 \nEXTLK,1,2 \nELDM,1,3 \nETRT,1,3 \nEXTLK,1,3 \nELDM,1,4 \nETRT,1,4 \nEXTLK,1,4 \n2 \nELDM,2,1 \nETRT,2,1 \nEXTLK,2,1 \nEDIR,2,2 \nERFT,2,2 \nESRM,2,2 \nELDM,2,3 \nETRT,2,3 \nEXTLK,2,3 \nELDM,2,4 \nETRT,2,4 \nEXTLK,2,4 \n3 \nELDM,3,1 \nETRT,3,1 \nEXTLK,3,1 \nELDM,3,2 \nETRT,3,2 \nEXTLK,3,2 \nEDIR,3,3 \nERFT,3,3 \nESRM,3,3 \nELDM,3,4 \nETRT,3,4 \nEXTLK,3,4 \n4 \nELDM,4,1 \nETRT,4,1 \nEXTLK,4,1 \nELDM,4,2 \nETRT,4,2 \nEXTLK,4,2 \nELDM,4,3 \nETRT,4,3 \nEXTLK,4,3 \nEDIR,4,4 \nERFT,4,4 \nESRM,4,4 \nReflection terms \nTransmission terms \nExamples SENS:CORR:CSET:DATA EXTLK,3,1 'cross talk between port 3 receiver \nand port 1 source. \nSENS:CORR:CSET:DATA ERSPT,1,1, \"a3/b4\" 'response tracking term \nfor ratioed measurement of port 4 test receiver over port 3 \nreference receiver. \n1693\n\nQuery Syntax SENSe<cnum>:CORRection:CSET:DATA? <eterm,portA, portB> \nReturn Type Block data \nDefault Not Applicable \nSENSe:CORRection:CSET:DELete <string> \n(Write-only) Deletes a Cal Set from the list of available Cal Sets. \nParameters \n<string> The GUID of the Cal Set to be deleted. The curly brackets and hyphens must \nbe included. Not case sensitive. \nExamples SENS:CORR:CSET:DEL '{2B893E7A-971A-11d5-8D6C-00108334AE96}' \nsense2:correction:cset:delete '{2B893E7A-971A-11d5-8D6C- \n00108334AE96}' \nQuery Syntax Not Applicable \nDefault Not Applicable \nSENSe<cnum>:CORRection:CSET:DESCription <string> \n(Read-Write) Sets or returns the descriptive string assigned to the selected Cal Set. Change this string \nso that you can easily identify each Cal Set. Apply and select the Cal Set using \nSENS:CORR:CSET:ACT. \nParameters \n<cnum> Any existing channel number. If unspecified, value is set to 1 \n<string> The descriptive string associated with the currently-selected Cal Set \nExamples SENS:CORR:CSET:DESC 'MyCalSet' \nsense2:correction:cset:description 'thisCalSet' \nQuery Syntax SENSe<cnum>:CORRection:CSET:DESCription? \nReturn Type String \nDefault Not Applicable \nSENSe<cnum>:CORRection:CSET:GUID <string> Superseded \n1694\n\nThis command is replaced by SENS:CORR:CSET:ACTivate. \n(Read-Write) Selects the Cal Set identified by the string parameter (GUID) and applies it to the \nspecified channel. \nA Cal Set cannot be selected for a channel which is not ON. \nIf the stimulus settings of the selected Cal Set differ from those of the selected channel, the instrument will \nautomatically change the channel's settings to match the Cal Set. \nParameters \n<cnum> Any existing channel number. If unspecified, value is set to 1 \n<string> GUID of the desired Cal Set. The curly brackets and hyphens must be included. \nExamples SENS:CORR:CSET:GUID '{2B893E7A-971A-11d5-8D6C-00108334AE96}' \nsense2:correction:cset:guid '{2B893E7A-971A-11d5-8D6C- \n00108334AE96}' \nQuery Syntax SENSe<cnum>:CORRection:CSET:GUID? \nReturns the GUID of the currently-selected Cal Set for the specified \nchannel. \nReturn Type String \nDefault Not Applicable \nSENSe<cnum>:CORRection:CSET:NAME <string> \n(Read-Write) Sets or queries the name of the Cal Set currently applied to the specified channel. \nParameters \n<cnum> Any existing channel number. If unspecified, value is set to 1 \n<string> Name of the Cal Set. Spaces or punctuation NOT allowed. \nExamples SENS:CORR:CSET:NAME 'MyCalSet' \nsense2:correction:cset:name 'thisCalSet' \nQuery Syntax SENSe<cnum>:CORRection:CSET:NAME? \nReturn Type String \nDefault Not Applicable \nSENSe<cnum>:CORRection:CSET[:SELect] <char> Superseded \n1695\n\nThis command is replaced by MMEM:LOAD \n(Read-Write) Restores a state file from memory. The file name is \"CSETx.cst\" where x is the user \nnumber assigned to <char>, and .cst specifies a cal set and instrument state. This is not the same \nsyntax as a file saved through the default choices from the front panel, which is \"at00x.cst\". For more \ninformation on the file naming syntax, see the MMEMory subsystem. Learn more about \nInstrument/Cal States. \nNote: This command does NOT select a Cal Set for a channel. To select a Cal Set, use \nSENS:CORR:CSET:ACTivate \nParameters \n<cnum> Any existing channel number. If unspecified, value is set to 1 \n<char> Choose from: \nDEF - Presets the analyzer \nUSER01 - Restores User01 calibration data \nUSER02 - Restores User02 calibration data \nthrough... \nUSER10 - Restores User10 calibration data \nExamples SENS:CORR:CSET DEF \nsense2:correction:cset:select user02 \nQuery Syntax SENSe<cnum>:CORRection:CSET[:SELect]? \nReturn Type Character \nDefault DEF \nSENSe<cnum>:CORRection:CSET:SAVE <char> \n1696\n\nThis command is NOT necessary after completion of a calibration. A Cal Set is automatically created, \napplied to the channel, and saved at the completion of a guided cal according to the preference setting \nSENS:CORR:PREF:CSET:SAVE. \n(Read Write) \nSaves the channel's Cal Set to the PNA hard drive. For example, use this command after writing data \nto a Cal Set using SENS:CORR:CSET:DATA (For Advanced Users). \nThe file name is saved as \"CSETx.cst\" where x is the user number assigned to <char>, and .cst \nspecifies a Cal Set and instrument state. This is not the same syntax as a file saved through the default \nchoices from the front panel, which is \"at00x.cst\". For more information on the file naming syntax, \nsee the MMEMory subsystem. Learn more about Instrument/Cal States. \nParameters \n<cnum> Any existing channel number. If unspecified, value is set to 1 \n<char> Choose from: \nUSER01 \nUSER02... \nUSER10 \nExamples SENS:CORR:CSET:SAVE USER03 \nsense2:correction:cset:save user09 \nQuery Syntax SENSe<cnum>:CORRection:CSET:SAVE? \nQueries the last correction set saved. \nReturn Type Character \nDefault Not applicable \nSENSe:CORRection:CSET:TSET:ALLPorts? <cset> \n1697\n\n(Read-only) Reads the port mapping used for the specified Cal Set. The returned values are the \nphysical ports. The POSITION of the returned values corresponds to the logical ports. \nFor example, with an N44xx test set, if the returned string is \"PNA 1,TS 2,PNA 2, TS 4\" this means: \nPNA 1 is assigned to logical port 1 \nTS 2 is assigned to logical port 2 \nPNA 2 is assigned to logical port 3 \nTS 4 is assigned to logical port 4 \nParameters \n<cset> (String) Name or GUID of the Cal Set. Use SENS:CORR:CSET:CAT? to read \nthe list of available Cal Set names or GUIDs. \nExamples SENS:CORR:CSET:TSET:ALLP? \"MyCalSet\" \nsens:correction:cset:tset:allports? \"{2B893E7A-971A-11d5-8D6C- \n00108334AE96}\" \nReturn Type String \nDefault Not Applicable \nSENSe:CORRection:CSET:TSET:TYPE? <cset> \n(Read-only) Reads the test set type (model) used for the specified Cal Set. \nParameters \n<cset> (String) Name or GUID of the Cal Set. Use SENS:CORR:CSET:CAT? to read \nthe list of available Cal Set names or GUIDs. \nExamples SENS:CORR:CSET:TSET:TYPE? \"MyCalSet\" \n'returns \"N44xx\" \nsens:correction:cset:tset:type? \"{2B893E7A-971A-11d5-8D6C- \n00108334AE96}\" \nReturn Type String \nDefault Not Applicable \nSENSe<ch>:CORRection:CSET:TYPE:CATalog? [format] \n1698\n\n(Read-only) Query the Cal Types available in the selected Cal Set. The output is a comma separated \nlist of Guids or a Cal Type names. Learn more about applying Cal Types using SCPI. \nUse CALC:CORR:TYPE to apply a Cal Type. \nParameters \n<ch> Any existing channel number. If unspecified, value is set to 1 \n[format] (Optional) Format of the output of cal types. choose from: \nNAME - (default) returns a list of cal type string names. \nGUID - returns a list of cal type GUIDs \nExamples SENS:CORR:CSET:TYPE:CAT? NAME \nSENS2:CORRection:CSET:TYPE:CAT? \nReturn Type String \nDefault Not Applicable \nLast modified: \n9/12/06 MQ Added TSET commands for multiport. \n1699\n\nSense:Correction:Extension Commands \nPerforms and applies Port Extensions. \nClick on a blue keyword to view the command details. \nSee Also \nExample Programs \nLearn about Port Extensions \nSynchronizing the PNA and Controller \nSCPI Command Tree \nSENSe<cnum>:CORRection:EXTension:AUTO:CONFig <char> \n(Read-Write) Sets the frequencies used to calculate Automatic Port Extension. Learn more about \ncalculating Automatic Port Extension. \nParameters \n<cnum> Any existing channel number. If unspecified, value is set to 1 \n<char> Frequencies to be used: \nCSPN Use current frequency span. \nAMKR - Use active marker frequency. \nUSPN - Use custom user span. Use SENS:CORR:EXT:AUTO:STAR and \nSENS:CORR:EXT:AUTO:STOP to specify start and stop frequency. \nExamples SENS:CORR:EXT:AUTO:CONF CSPN \nsense2:correction:extension:auto:config amkr \nQuery Syntax SENSe<cnum>:CORRection:EXTension:AUTO:CONFig ? \n1700\n\nReturn Type Character \nDefault CSPN \nSENSe<cnum>:CORRection:EXTension:AUTO:DCOFfset <bool> \n(Read-Write) Specifies whether or not to include DC Offset as part of automatic port extension. Learn \nmore about Automatic DC Offset. Only allowed when SENS:CORR:EXT:AUTO:LOSS is set to ON. \nParameters \n<cnum> Any existing channel number. If unspecified, value is set to 1 \n<bool> ON (or 1) - Includes DC Offset correction. \n
